vi "BrakeSwitchCommander.vi"(8 "CurrentTick":dbl, 9 "TickMemoryIn":dbl, 10 "BrakeStateOld":bool, 11 "BrakeStateNew":bool) -> (2 "TickMemoryOut":dbl, 3 "BrakeSwitch Control":bool)   [LabVIEW 2019]
panel:
  # "This VI is used to activate the BrakeSwitch Resistor (to prevent brake overheat, it reduces the voltage sent to motor breaks) only 1sec after the brake has been activated.\nin this way we allow one second for the brake to open properly at max power (24V), before switching to power saving (16V)"
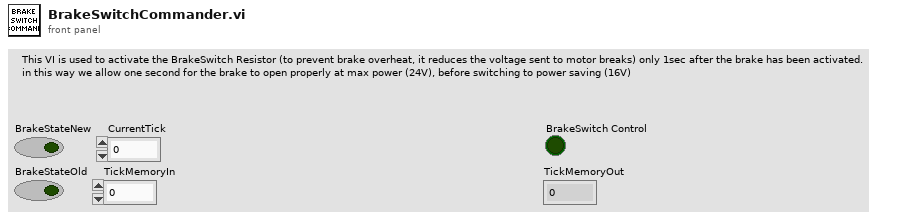
[diagram p1: front panel]
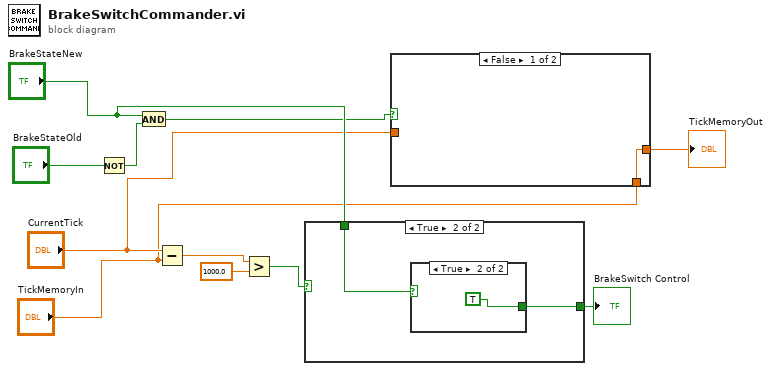
[diagram p0: block diagram]
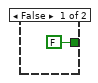
[diagram p3: hidden frame]
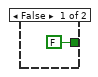
[diagram p4: hidden frame]
diagram:
  n1 = Not(x="BrakeStateOld") -> (.not. x?=w10:bool)
  n2 = And(x="BrakeStateNew", y=w10) -> (x .and. y?=w5:bool)
  n3 = Subtract(x="CurrentTick", y="TickMemoryIn") -> (x-y=w9:dbl)
  n4 = Greater?(x=w9, y=1000.0) -> (0:w7:bool)
  n5 = case shown="True" w7 {
    tunnel: "BrakeStateNew" -> [_ w14]
    tunnel: [FALSE ("BrakeStateNew 2") w13] -> w1
    frame False {
    }
    frame True {
      n6 = case shown="True" w14 {
        tunnel: [FALSE ("BrakeStateNew 2") TRUE ("BrakeStateNew 2")] -> w13
        frame False {
        }
        frame True {
        }
      }
    }
  }
  "BrakeSwitch Control" <- w1
  n7 = case shown="False" w5 {
    tunnel: "CurrentTick" -> [_ w18]
    tunnel: [w17 w18] -> w3
    tunnel: "TickMemoryIn" -> [w17 _]
    frame False {
    }
    frame True {
    }
  }
  "TickMemoryOut" <- w3
